vi "HEAD_req_PS.vi"(7 "Headers":string, 8 "error in":errorcluster, 11 "URL":string) -> (0 "error out":errorcluster, 3 "HEAD Request":string)   [LabVIEW 2016, in "Request.lvclass"]
uses:
  Object Oriented Version/Request.lvclass
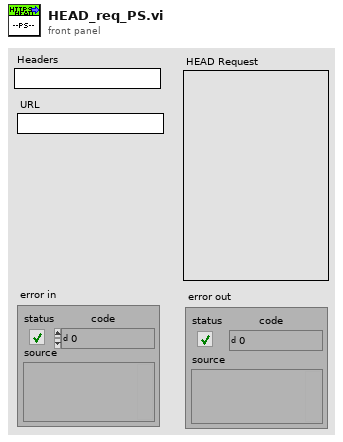
[diagram p1: front panel]
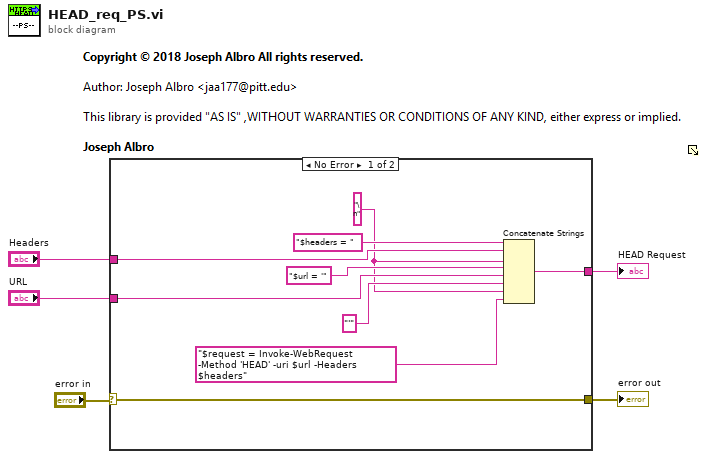
[diagram p0: block diagram]
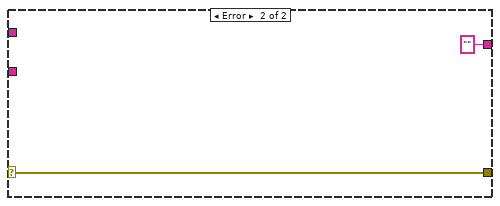
[diagram p2: hidden frame]
diagram:
  n1 = case shown="No Error" "error in" {
    selector: "error in" -> [w6 w15]
    tunnel: "Headers" -> [w14 _]
    tunnel: "URL" -> [w11 _]
    tunnel: [w9 ""] -> w3
    tunnel: [w6 w15] -> w1
    frame No Error {
      w8 = "\n"
      n2 = Concatenate Strings("$headers = ", w14, w8, "$url = '" ("string"), w11, "'" ("string"), w8, "$request = Invoke-WebRequest -Method 'HEAD' -uri $url -Headers $headers" ("string")) -> (w9:string)
    }
    frame Error {
    }
  }
  "HEAD Request" <- w3
  "error out" <- w1
